vi "Read_Dwld_DataBase.vi"(4 "error in (no error)":errorcluster, 7 "Select Table Name":string="Bar_LIV") -> (0 "error out":errorcluster={"status"=TRUE, "code"=-2147217865, "source"="NI_Database_API.lvlib:Conn Execute.vi->NI_Database_API.lvlib:DB Tools Select Data.vi->Read_Dwld_DataBase.vi<ERR>ADO Error: 0x80040E37\r\nException occured in Microsoft OLE DB Provider for ODBC Drivers: [Microsoft][ODBC SQL Server Driver][SQL Server]Invalid object name 'dbo_Bar_LIV'. in NI_Database_API.lvlib:Conn Execute.vi->NI_Database_API.lvlib:DB Tools Select Data.vi->Read_Dwld_DataBase.vi"}, 1 "Column Info":string[](array[string]), 2 "Output Data":string[][](array[string]), 3 "Output selection string":string[][](array[string]))   [LabVIEW 2017]
uses:
  <vilib>/addons/database/Connection.llb/DB Tools Open Connec (String).vi
  <vilib>/addons/database/_DB Variant To Data/Database Variant To Data.xnode
  <vilib>/addons/database/NI_Database_API.lvlib
panel:
  out "Output selection subarry":string[][](array[string])
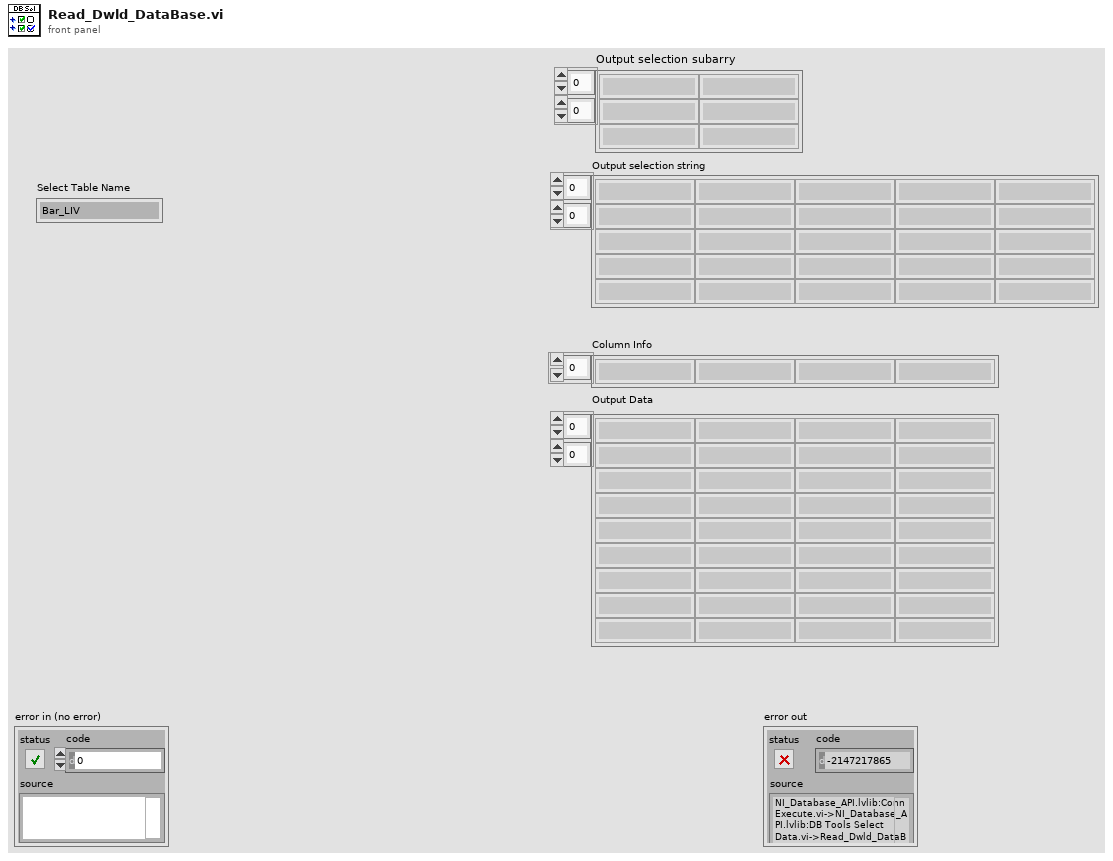
[diagram p1: front panel]
types:
  T1 = typedef "NI_Database_API.lvlib/Conn ObjectReference.ctl" = refnum<k1>
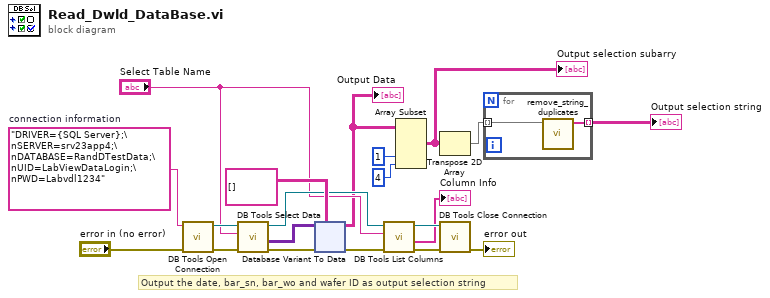
[diagram p0: block diagram]
diagram:
  w20 = "DRIVER={SQL Server};\nSERVER=srv23app4;\nDATABASE=RandDTestData;\nUID=LabViewDataLogin;\nPWD=Labvdl1234"  # connection information
  # "Output the date, bar_sn, bar_wo and wafer ID as output selection string"
  n1 = call-poly <vilib>:"DB Tools Open Connection.vi"("error in (no error)"="error in (no error)", "connection information"=w20) -> ("error out"=w17:errorcluster, "connection reference"=w18:T1)  [unwired: 6 in]
  n2 = call <vilib>:"DB Tools Select Data.vi"("error in (no error)"=w17, "table"="Select Table Name", "connection reference"=w18) -> ("error out"=w14:errorcluster, "data"=w15:variant[][], "connection reference out"=w12:T1)  [unwired: 3 in]
  n3 = xnode "Database Variant To Data"("database variant"=w15, "error in (no error)"=w14, "type"=string[][] []) -> ("data"=w6:string[][], "error out"=w11:errorcluster)
  "Output Data" <- w6
  n4 = call <vilib>:"DB Tools List Columns.vi"("error in (no error)"=w11, "table"="Select Table Name", "connection reference"=w12) -> ("error out"=w10:errorcluster, "columns"=→"Column Info":string[], "connection reference out"=w9:T1)  [unwired: 1 in, 1 out]
  n5 = Array Subset(array=w6, index (col)=1 ("index"), length (col)=4 ("length")) -> (w3:string[][])  [unwired: 2 in]
  "Output selection subarry" <- w3
  n6 = Transpose 2D Array(2D array=w3) -> (transposed array=w2:string[][])
  n7 = call <vilib>:"DB Tools Close Connection.vi"("error in (no error)"=w10, "connection reference"=w9) -> ("error out"=→"error out":errorcluster)  [unwired: 5 in]
  n8 = for {
    tunnel: w2 -> [w21] mode=indexing
    tunnel: [w22] -> w1 mode=indexing
    n9 = call "remove_string_duplicates.vi"("In"=w21) -> ("Out"=w22:string[])  [unwired: 10 in]
  }
  "Output selection string" <- w1
